vi "Append Control Info to Report.vi"(0 "report in":refnum<class "NI_report.lvclass">, 1 "level":i32, 5 "ctl refnum":refnum<vi>, 7 "alignment (default)":T2, 9 "image format (jpeg)":enum32{"PNG", "JPEG", "GIF"}(ring), 11 "error in":errorcluster, 12 "include control descriptions?":bool, 13 "include control datatype information?":bool, 14 "MS Office parameters":T1) -> (4 "report out":refnum<class "NI_report.lvclass">, 8 "start out (word)":i32, 10 "end out (word)":i32, 15 "error out":errorcluster)   [LabVIEW 2017, in "NI_ReportGenerationCore.lvlib"]
uses:
  <vilib>/Utility/NIReport.llb/NI_ReportGenerationCore.lvlib
  <vilib>/Utility/NIReport.llb/NI_report.lvclass
  <vilib>/Utility/NIReport.llb/HTML Report Image Alignment.ctl
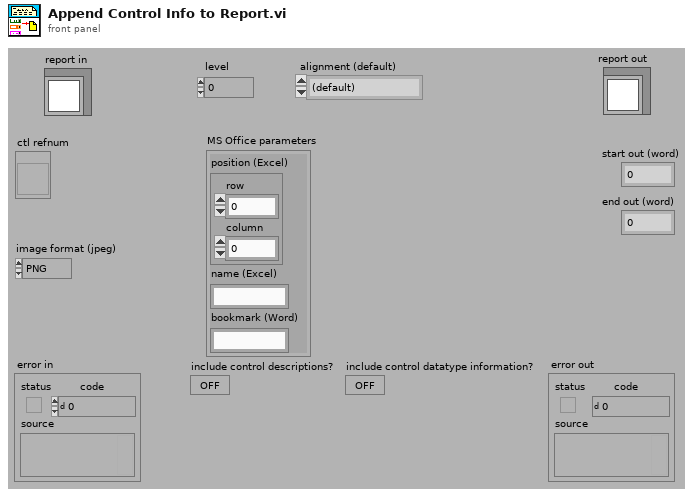
[diagram p1: front panel]
types:
  T1 = cluster{"position (Excel)":cluster{"row":i32, "column":i32}, "name (Excel)":string, "bookmark (Word)":string}
  T2 = typedef "NI_ReportGenerationCore.lvlib/HTML Report Image Alignment.ctl" = enum16{"(default)", "LEFT", "RIGHT", "TOP", "TEXTTOP", "MIDDLE", "ABSMIDDLE", "BASELINE", "BOTTOM", "ABSBOTTOM"}
  T3 = typedef "imagedata.ctl" = cluster{"image type":i32, "image depth":i32, "image":u8[], "mask":u8[], "colors":u32[], "Rectangle":cluster{"left":i16, "top":i16, "right":i16, "bottom":i16}}
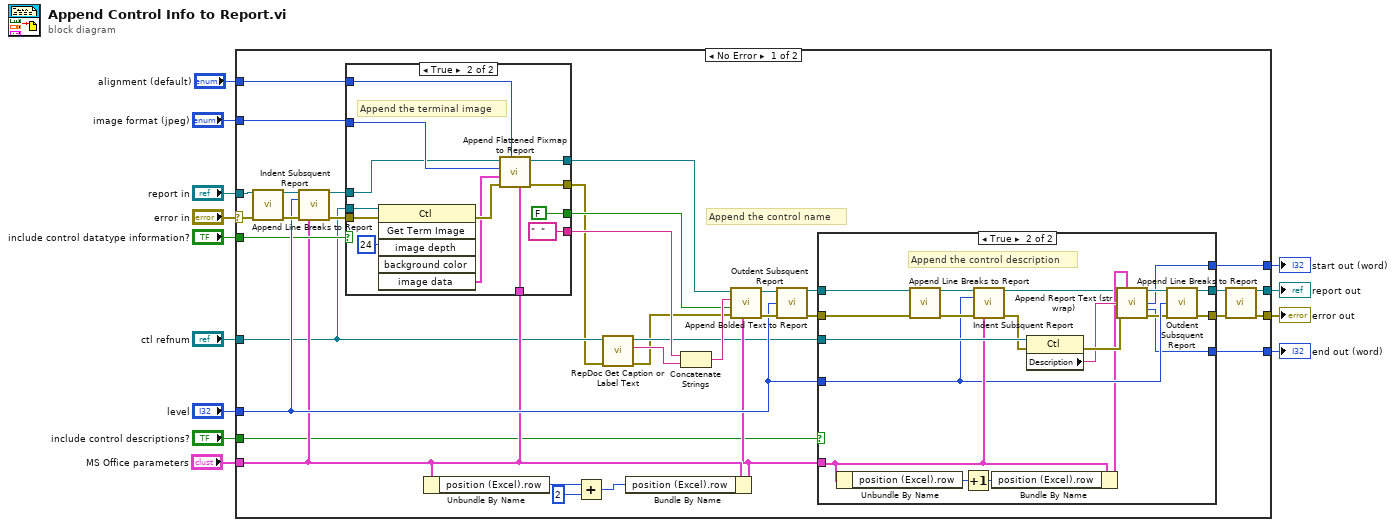
[diagram p0: block diagram]
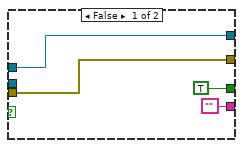
[diagram p3: hidden frame]
diagram:
  n1 = case shown="No Error" "error in" {
    selector: "error in" -> [w24 w88]
    tunnel: "ctl refnum" -> [w21 _]
    tunnel: "image format (jpeg)" -> [w48 _]
    tunnel: [w47 w89] -> w11
    tunnel: [w40 w88] -> w10
    tunnel: "include control descriptions?" -> [w22 _]
    tunnel: "report in" -> [w38 w89]
    tunnel: "level" -> [w34 _]
    tunnel: "alignment (default)" -> [w33 _]
    tunnel: "include control datatype information?" -> [w32 _]
    tunnel: "MS Office parameters" -> [w31 _]
    tunnel: [w26 _] -> w3
    tunnel: [w25 _] -> w2
    frame No Error {
      # "Append the control name"
      n2 = call <vilib>:"Append Line Breaks to Report.vi"("report in"=w38, "error in (no error)"=w24) -> ("report out"=w39:refnum<class "NI_report.lvclass">, "error out"=w37:errorcluster)  [unwired: 12 in]
      n3 = call-dynamic "Indent Subsquent Report.vi"("report in"=w39, "level"=w34, "error in (no error)"=w37, "MS Office parameters"=w31) -> ("report out"=w14:refnum<class "NI_report.lvclass">, "error out"=w36:errorcluster)  [unwired: 10 in]
      n4 = case shown="True" w32 {
        tunnel: [w71 w83] -> w43
        tunnel: w36 -> [w74 w81]
        tunnel: [w74 w82] -> w17
        tunnel: [TRUE ("On new line?") FALSE ("On new line?")] -> w44
        tunnel: ["" "  "] -> w46
        tunnel: w48 -> [_ w84]
        tunnel: w21 -> [_ w86]
        tunnel: w31 -> [_ w80]
        tunnel: w33 -> [_ w79]
        tunnel: w14 -> [w71 w75]
        frame False {
        }
        frame True {
          # "Append the terminal image"
          n5 = invoke class="Ctl" method="Get Term Image"(reference=w86, error in=w81, "image depth"=24) -> (error out=w85:errorcluster, "image data"=w78:T3)  [unwired: 3 in, 4 out]
          n6 = call <vilib>:"Append Flattened Pixmap to Report.vi"("MS Office parameters"=w80, "alignment (default)"=w79, "error in (no error)"=w85, "image data"=w78, "image format (jpeg)"=w84, "report in"=w75) -> ("error out"=w82:errorcluster, "report out"=w83:refnum<class "NI_report.lvclass">)  [unwired: 2 in, 2 out]
        }
      }
      n7 = Unbundle By Name(w31) -> ("position (Excel).row"=w28:i32)
      n8 = Add(x=w28, y=2) -> (x+y=w29:i32)
      n9 = call <vilib>:"RepDoc Get Caption or Label Text.vi"("error in (no error)"=w17, "Ctl Refnum"=w21) -> ("error out"=w18:errorcluster, "Caption or Label"=w19:string, "Ctl Refnum out"=w20:refnum<vi>)  [unwired: 7 in]
      n10 = Bundle By Name(cluster=w31, "position (Excel).row"=w29) -> (w30:T1)
      n11 = Concatenate Strings(w46, w19) -> (w45:string)
      n12 = call <vilib>:"Append Bolded Text to Report.vi"("MS Office parameters"=w30, "error in"=w18, "On new line?"=w44, "Text"=w45, "report in"=w43) -> ("error out"=w35:errorcluster, "report out"=w16:refnum<class "NI_report.lvclass">)  [unwired: 2 out]
      n13 = call-dynamic "Outdent Subsquent Report.vi"("report in"=w16, "level"=w34, "error in (no error)"=w35) -> ("report out"=w15:refnum<class "NI_report.lvclass">, "error out"=w23:errorcluster)  [unwired: 11 in]
      n14 = case shown="True" w22 {
        tunnel: w23 -> [w50 w68]
        tunnel: w15 -> [w49 w69]
        tunnel: [w50 w65] -> w42
        tunnel: [w49 w59] -> w41
        tunnel: w20 -> [_ w70]
        tunnel: w34 -> [_ w61]
        tunnel: w30 -> [_ w63]
        tunnel: [_ w53] -> w26
        tunnel: [_ w54] -> w25
        frame False {
        }
        frame True {
          # "Append the control description"
          n15 = Unbundle By Name(w63) -> ("position (Excel).row"=w64:i32)
          n16 = call <vilib>:"Append Line Breaks to Report.vi"("report in"=w69, "error in (no error)"=w68) -> ("report out"=w51:refnum<class "NI_report.lvclass">, "error out"=w67:errorcluster)  [unwired: 12 in]
          n17 = Increment(x=w64) -> (x+1=w62:i32)
          n18 = call-dynamic "Indent Subsquent Report.vi"("report in"=w51, "level"=w61, "error in (no error)"=w67, "MS Office parameters"=w63) -> ("report out"=w52:refnum<class "NI_report.lvclass">, "error out"=w66:errorcluster)  [unwired: 10 in]
          n19 = Bundle By Name(cluster=w63, "position (Excel).row"=w62) -> (w55:T1)
          n20 = property class="Ctl"(reference=w70, error in=w66) -> (error out=w57:errorcluster, "Description"=w56:string)  [unwired: 1 out]
          n21 = call <vilib>:"Append Report Text (str wrap).vi"("report in"=w52, "MS Office parameters"=w55, "text"=w56, "error in (no error)"=w57) -> ("report out"=w60:refnum<class "NI_report.lvclass">, "start out (Word)"=w53:i32, "end out (Word)"=w54:i32, "error out"=w58:errorcluster)  [unwired: 8 in]
          n22 = call-dynamic "Outdent Subsquent Report.vi"("report in"=w60, "level"=w61, "error in (no error)"=w58) -> ("report out"=w59:refnum<class "NI_report.lvclass">, "error out"=w65:errorcluster)  [unwired: 11 in]
        }
      }
      n23 = call <vilib>:"Append Line Breaks to Report.vi"("report in"=w41, "error in (no error)"=w42) -> ("report out"=w47:refnum<class "NI_report.lvclass">, "error out"=w40:errorcluster)  [unwired: 12 in]
    }
    frame Error {
    }
  }
  "report out" <- w11
  "error out" <- w10
  "start out (word)" <- w3
  "end out (word)" <- w2
